vi "Capacitance PID.vi"() -> ()   [LabVIEW 2024]
doc: "This VI is meant to be used with the process control package (PID controller) and an MIO-series or Lab-PC data acquisition board. Connect the analog output to the analog input through the resistor-capacitor network shown on the front panel (scroll down to view it). The VI attempts to adjust the analog output so that the input (process variable or PV) equals the setpoint (SP). SP and PV are displayed on a strip chart. You can experiment with different controller tuning methods and try for the fastest settling time with the least overshoot.\n\nThe input span is -10 to +10 V, or 20V = 100%. The output span is 0 to +10 V, or 10V = 100%. PV and SP are in Volts. Your MIO board should be set up for differential input and -10 to +10 V range; the output should be unipolar, 10V (these are all factory defaults). If you elect to use other settings, run the configuration VIs as necessary.\n\nThe recommended network has a DC gain of 0.33, an effective deadtime of about 5 Sec., and an effective time constant of about 30 Sec."
uses:
  <vilib>/addons/control/pid/NI_PID__autopid compat.lvlib
  <vilib>/_DAQmxBase/Internals/DAQmxBase Create Channel (AO-Voltage-Basic).vi
  <vilib>/Utility/error.llb/DialogType.ctl
  <vilib>/_DAQmxBase/Internals/DAQmxBase Write (Analog 1D DBL NChan 1Samp).vi
panel:
  out "Ccyle #":i32
  in  "Bias":dbl format="%.2f"
  in  "gain scheduling":T1={"gain schedule"=[40.0, 70.0, 100.0], "PID parameters"=[{"Kc"=20.0, "Ti (min)"=0.008, "Td (min)"=0.006}, {"Kc"=20.0, "Ti (min)"=0.008, "Td (min)"=0.006}, {"Kc"=20.0, "Ti (min)"=0.008, "Td (min)"=0.006}], "scheduling input"=0} {"scheduling input" items=["Setpoint", "Process variable", "Controller output", "Gain scheduling input"]; "PID parameters"."Td (min)" format="%.4f"; "PID parameters"."Ti (min)" format="%.4f"; "gain schedule" format="%.2f"}
  in  "?":bool
  in  "options":T2={"sp low"=-10.0, "sp high"=10.0, "out low"=0.0, "out high"=10.0, "hold (F)"=FALSE, "auto (T)"=TRUE, "pro. band (F)"=FALSE, "reverse acting (T)"=TRUE, "beta"=1.0, "linearity"=1.0, "dt (s)"=-1.0} {"dt (s)" format="%.2f"; "linearity" min=0.0 max=1.0 format="%.2f"; "sp low" format="%.2f"; "sp high" format="%.2f"; "out low" format="%.2f"; "out high" format="%.2f"; "beta" min=0.0 max=1.0 format="%.2f"}
  in  "STOP":bool
  in  "Setpoint (V)":dbl(slide)=0.5 min=0.0 max=1.0 step=0.0001 scale=0.9..1.0 scale format="%.2f"
  out "Output (V)":dbl(slide) scale=0.0..10.0 scale format="%.2f"
  in  "Cycle Time (sec)":dbl=0.5 format="%.2f"
  in  "Manual Out (V)":dbl(knob) scale=-2.0..10.0
  out "Trend":cluster{dbl, "Setpoint (V)":dbl}(graph)
  # "SP & PV range:"
  # "Output range:"
  # "-1: default,using\nsystem clock"
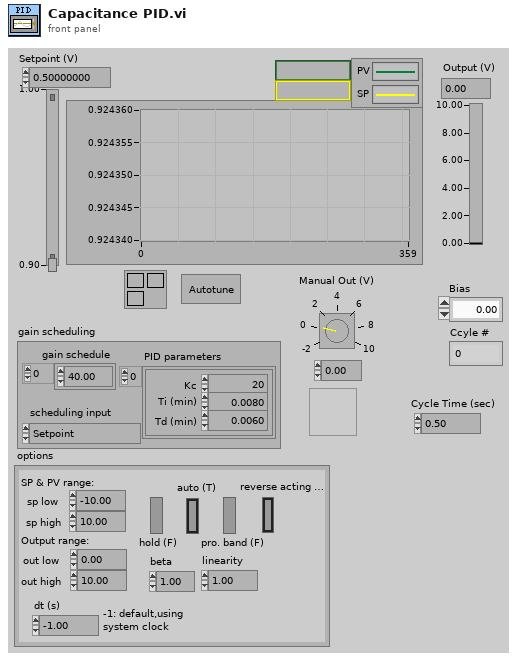
[diagram p1: front panel]
types:
  T1 = cluster{"gain schedule":dbl[], "PID parameters":cluster{"Kc":dbl, "Ti (min)":dbl, "Td (min)":dbl}[], "scheduling input":u16}
  T2 = cluster{"sp low":dbl, "sp high":dbl, "out low":dbl, "out high":dbl, "hold (F)":bool, "auto (T)":bool, "pro. band (F)":bool, "reverse acting (T)":bool, "beta":dbl, "linearity":dbl, "dt (s)":dbl}
  T3 = typedef "DialogType.ctl" = u16
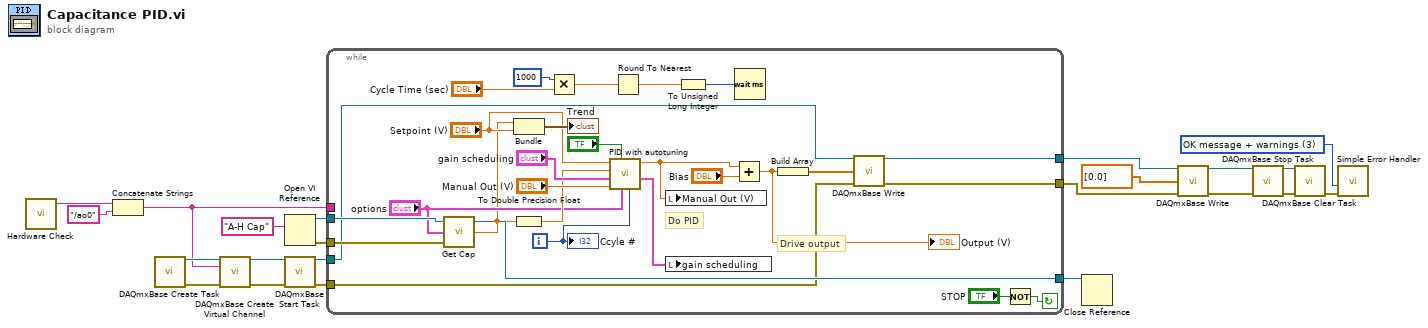
[diagram p0: block diagram]
diagram:
  w11 = T3 3 items=["no dialog", "OK message", "continue or stop message", "OK message + warnings", "continue/stop + warnings"] ("type of dialog (OK msg:1)")
  n1 = call "Hardware Check.vi"() -> ("Data Acq Device"=w19:string)  [unwired: 1 in, 2 out]
  n2 = Concatenate Strings(w19, "/ao0" ("string")) -> (w12:string)
  n3 = call <vilib>:"DAQmxBase Create Task.vi"() -> ("task out"=w13:refnum<k21>, "error out"=w14:errorcluster)  [unwired: 14 in]
  n4 = call-poly <vilib>:"DAQmxBase Create Virtual Channel.vi"("task in"=w13, "physical channels"=w12, "error in"=w14) -> ("task out"=w15:refnum<k21>, "error out"=w16:errorcluster)  [unwired: 11 in]
  n5 = Open VI Reference(vi path="A-H Cap") -> (vi reference=w21:refnum<vi>, error out=w18:errorcluster)  [unwired: 5 in]
  n6 = call <vilib>:"DAQmxBase Start Task.vi"("task/channels in"=w15, "error in"=w16) -> ("task out"=w4:refnum<k21>, "error out"=w3:errorcluster)  [unwired: 12 in]
  n7 = while {
    tunnel: w18 -> [w35]
    tunnel: [w37] -> w20
    tunnel: w21 -> [w38]
    tunnel: w12 -> [_]
    tunnel: w4 -> [w27]
    tunnel: w3 -> [w26]
    tunnel: [w25] -> w2
    tunnel: [w24] -> w1
    i -> [w43]
    stop <- w49 continue-if-true
    # "Do PID"
    # "Drive output"
    n8 = call "Get Cap.vi"("error in"=w35, "options"="options", "VI Refnum 2"=w38) -> ("Setpoint (V)"=w33:dbl, "VI Refnum"=w37:refnum<vi>)  [unwired: 1 in]
    n9 = Bundle("Setpoint (V)"=w33, "Setpoint (V)"="Setpoint (V)") -> (→"Trend":cluster{"Setpoint (V)":dbl, "Setpoint (V)":dbl})  [unwired: 1 in]
    n10 = To Double Precision Float(number=w33) -> (double precision float=w39:dbl)
    n11 = Multiply(x=1000, y="Cycle Time (sec)") -> (x*y=w46:dbl)
    n12 = call <vilib>:"PID with autotuning.vi"("iteration"=w43, "options"="options", "autotune? (F)"="?", "manual control"="Manual Out (V)", "gain scheduling"="gain scheduling", "process variable"=w39, "setpoint"="Setpoint (V)") -> ("updated parameters"=w42:T1, "output"=w30:dbl)  [unwired: 2 in, 1 out]
    n13 = Round To Nearest(number=w46) -> (nearest integer value=w29:dbl)
    n14 = local write "Manual Out (V)"(w30) -> ()
    n15 = local write "gain scheduling"(w42) -> ()
    n16 = To Unsigned Long Integer(number=w29) -> (unsigned 32bit integer=w28:u32)
    n17 = Add(x=w30, y="Bias") -> (x+y=w31:dbl)
    "Output (V)" <- w31
    n18 = Wait (ms)(milliseconds to wait=w28) -> ()  [unwired: 1 out]
    n19 = Build Array(w31) -> (w23:dbl[])
    n20 = call-poly <vilib>:"DAQmxBase Write.vi"("task/channels in"=w27, "data"=w23, "error in"=w26) -> ("task out"=w24:refnum<k21>, "error out"=w25:errorcluster)  [unwired: 10 in, 1 out]
    n21 = Not(x="STOP") -> (.not. x?=w49:bool)
    "Ccyle #" <- w43
  }
  n22 = Close Reference(reference=w20) -> ()  [unwired: 1 in, 1 out]
  n23 = call-poly <vilib>:"DAQmxBase Write.vi"("task/channels in"=w1, "data"=dbl[] [0.0], "error in"=w2) -> ("task out"=w6:refnum<k21>, "error out"=w7:errorcluster)  [unwired: 10 in, 1 out]
  n24 = call <vilib>:"DAQmxBase Stop Task.vi"("task/channels in"=w6, "error in"=w7) -> ("task out"=w8:refnum<k21>, "error out"=w9:errorcluster)  [unwired: 12 in]
  n25 = call <vilib>:"DAQmxBase Clear Task.vi"("task in"=w8, "error in"=w9) -> ("error out"=w10:errorcluster)  [unwired: 13 in]
  n26 = call <vilib>:"Simple Error Handler.vi"("type of dialog (OK msg:1)"=w11, "error in (no error)"=w10) -> ()  [unwired: 3 in, 5 out]
